vi "convert_string_to_doubleArray.vi"(2 "Max Elements Count (All)":i32=-1, 3 "default (0)":dbl, 4 "string in":string) -> (0 "double array size out":i32, 1 "double array out":dbl[](array[numeric]))   [LabVIEW 2020, in "Rohde&Schwarz RTx Oscilloscopes.lvlib" / "rsidr_core.lvlib"]
uses:
  rsidr_core.lvlib
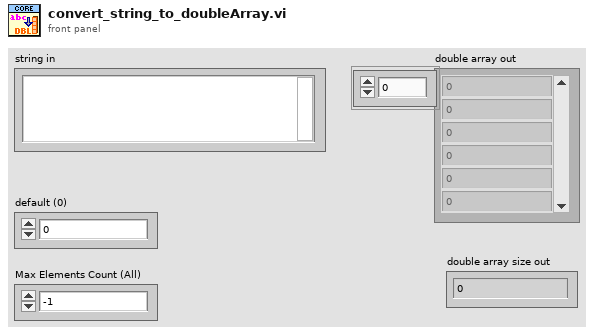
[diagram p1: front panel]
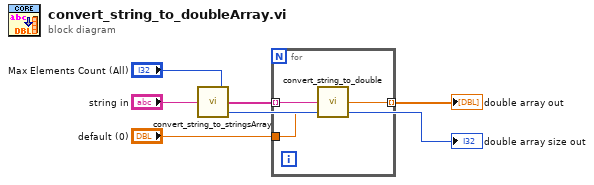
[diagram p0: block diagram]
diagram:
  n1 = call "convert_string_to_stringsArray.vi"("Max Elements Count (All)"="Max Elements Count (All)", "String in"="string in") -> ("string array size out"=→"double array size out":i32, "string array out"=w5:string[])  [unwired: 2 in]
  n2 = for {
    tunnel: w5 -> [w9] mode=indexing
    tunnel: "default (0)" -> [w8]
    tunnel: [w7] -> w3 mode=indexing
    n3 = call "convert_string_to_double.vi"("default (0)"=w8, "String in"=w9) -> ("double value out"=w7:dbl)  [unwired: 3 in]
  }
  "double array out" <- w3
